vi "Arm Constants.vi"() -> ()   [LabVIEW 2018]
panel:
  in  "Encoder Counts per Degree":dbl=40.0
  in  "Center Turret to Edge":dbl=20.5
  in  "Intake Length":dbl=20.5
  in  "Forearm Length":dbl=39.0
  in  "Bicep Length":dbl=35.5
  in  "Turret Height":dbl=9.75
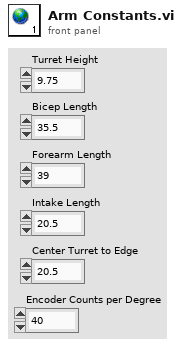
[diagram p1: front panel]
diagram:
